vi "力特性判定.vi"(0 "曲线引用":refnum<vi>, 1 "力特性判定条件":T1, 3 "错误输入":errorcluster) -> (7 "曲线引用输出":refnum<vi>, 8 "OK？":bool, 10 "错误输出":errorcluster)   [LabVIEW 2020]
uses:
  Global_Variable/A131258.vi
  Global_Variable/Global.vi
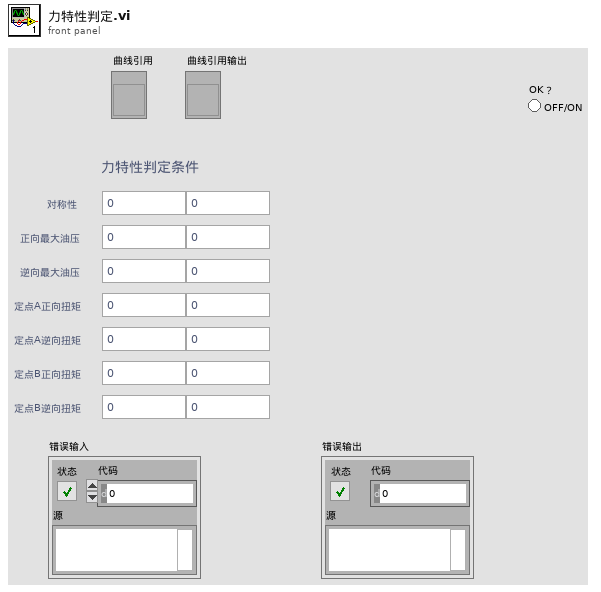
[diagram p1: front panel]
types:
  T1 = cluster{"           对称性":cluster{"下限":dbl, "上限":dbl}, "  正向最大油压":cluster{"下限":dbl, "上限":dbl}, "  逆向最大油压":cluster{"下限":dbl, "上限":dbl}, "定点A正向扭矩":cluster{"下限":dbl, "上限":dbl}, "定点A逆向扭矩":cluster{"下限":dbl, "上限":dbl}, "定点B正向扭矩":cluster{"下限":dbl, "上限":dbl}, "定点B逆向扭矩":cluster{"下限":dbl, "上限":dbl}}
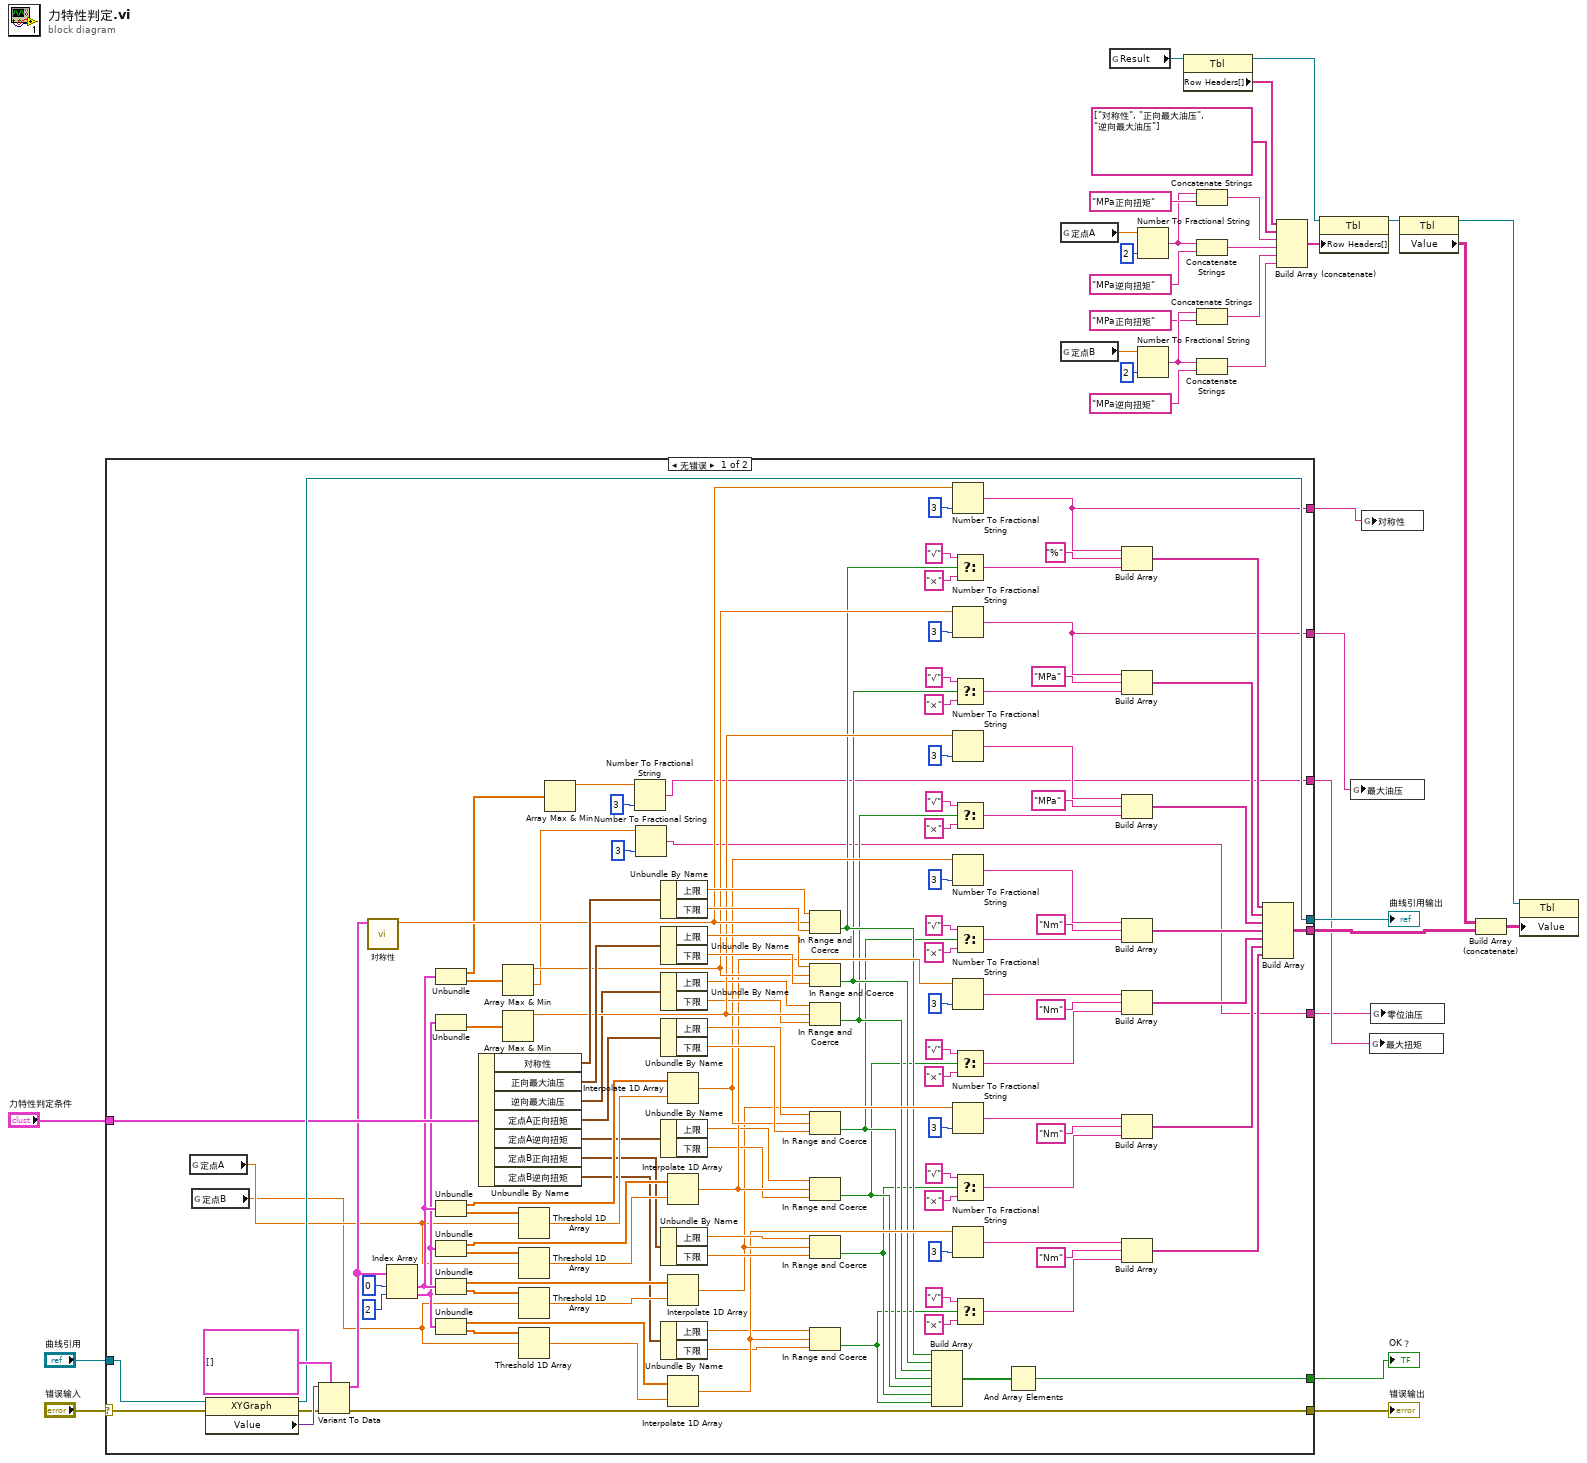
[diagram p0: block diagram]
diagram:
  n1 = case shown="无错误" "错误输入" {
    selector: "错误输入" -> [w155 w159]
    tunnel: [w152 w159] -> w33
    tunnel: "曲线引用" -> [w151 w158]
    tunnel: [w154 w158] -> w31
    tunnel: [w49 _] -> w30
    tunnel: "力特性判定条件" -> [w150 _]
    tunnel: [w48 _] -> w25
    tunnel: [w43 _] -> w4
    tunnel: [w42 _] -> w3
    tunnel: [w38 _] -> w2
    tunnel: [w35 _] -> w1
    frame No Error {
      n2 = global read "A131258.vi" "定点A"() -> (w45:dbl)
      n3 = global read "A131258.vi" "定点B"() -> (w44:dbl)
      n4 = property class="XYGraph"(reference=w151, error in=w155) -> (reference out=w154:refnum<vi>, error out=w153:errorcluster, "Value"=w157:variant)
      n5 = Variant To Data(error in=w153, type=cluster{dbl[], dbl[]}[] [], Variant=w157) -> (data=w140:cluster{dbl[], dbl[]}[], error out=w152:errorcluster)
      n6 = call "对称性.vi"("XY图"=w140) -> ("对称性"=w146:dbl)  [unwired: 10 in]
      n7 = Index Array(array=w140, index #1=0 ("索引"), index #2=2 ("索引")) -> (element #1=w79:cluster{dbl[], dbl[]}, element #2=w66:cluster{dbl[], dbl[]})
      n8 = Unbundle(w79) -> (w41:dbl[], w47:dbl[])
      n9 = Unbundle(w66) -> (w46:dbl[])  [unwired: 1 out]
      n10 = Unbundle(w79) -> (w111:dbl[], w112:dbl[])
      n11 = Unbundle(w66) -> (w105:dbl[], w104:dbl[])
      n12 = Unbundle(w79) -> (w85:dbl[], w86:dbl[])
      n13 = Unbundle(w66) -> (w76:dbl[], w75:dbl[])
      n14 = Unbundle By Name(w150) -> ("对称性"=w149:cluster{"下限":dbl, "上限":dbl}, "正向最大油压"=w132:cluster{"下限":dbl, "上限":dbl}, "逆向最大油压"=w121:cluster{"下限":dbl, "上限":dbl}, "定点A正向扭矩"=w108:cluster{"下限":dbl, "上限":dbl}, "定点A逆向扭矩"=w95:cluster{"下限":dbl, "上限":dbl}, "定点B正向扭矩"=w80:cluster{"下限":dbl, "上限":dbl}, "定点B逆向扭矩"=w65:cluster{"下限":dbl, "上限":dbl})
      n15 = Array Max & Min(array=w47) -> (max value=w131:dbl, min value=w36:dbl)  [unwired: 2 out]
      n16 = Array Max & Min(array=w46) -> (max value=w130:dbl)  [unwired: 3 out]
      n17 = Threshold 1D Array(2:w45, 3:w112) -> (0:w110:dbl)  [unwired: 1 in]
      n18 = Threshold 1D Array(2:w45, 3:w104) -> (0:w106:dbl)  [unwired: 1 in]
      n19 = Threshold 1D Array(2:w44, 3:w86) -> (0:w84:dbl)  [unwired: 1 in]
      n20 = Threshold 1D Array(2:w44, 3:w75) -> (0:w77:dbl)  [unwired: 1 in]
      n21 = Array Max & Min(array=w41) -> (max value=w39:dbl)  [unwired: 3 out]
      n22 = Number To Fractional String(number=w39, precision (6)=i16 3 ("精度(6)")) -> (F-format string=w38:string)  [unwired: 2 in]
      n23 = Number To Fractional String(number=w36, precision (6)=i16 3 ("精度(6)")) -> (F-format string=w35:string)  [unwired: 2 in]
      n24 = Unbundle By Name(w149) -> ("上限"=w148:dbl, "下限"=w147:dbl)
      n25 = Unbundle By Name(w132) -> ("上限"=w133:dbl, "下限"=w134:dbl)
      n26 = Unbundle By Name(w121) -> ("上限"=w129:dbl, "下限"=w128:dbl)
      n27 = Unbundle By Name(w108) -> ("上限"=w113:dbl, "下限"=w114:dbl)
      n28 = Unbundle By Name(w95) -> ("上限"=w103:dbl, "下限"=w102:dbl)
      n29 = Unbundle By Name(w80) -> ("上限"=w87:dbl, "下限"=w88:dbl)
      n30 = Unbundle By Name(w65) -> ("上限"=w74:dbl, "下限"=w73:dbl)
      n31 = Interpolate 1D Array(1:w110, 2:w111) -> (0:w109:dbl)
      n32 = Interpolate 1D Array(1:w106, 2:w105) -> (0:w107:dbl)
      n33 = Interpolate 1D Array(1:w84, 2:w85) -> (0:w83:dbl)
      n34 = Interpolate 1D Array(1:w77, 2:w76) -> (0:w78:dbl)
      n35 = In Range and Coerce(upper limit=w148, x=w146, lower limit=w147) -> (In Range?=w63:bool)  [unwired: 1 out]
      n36 = In Range and Coerce(upper limit=w133, x=w131, lower limit=w134) -> (In Range?=w61:bool)  [unwired: 1 out]
      n37 = In Range and Coerce(upper limit=w129, x=w130, lower limit=w128) -> (In Range?=w59:bool)  [unwired: 1 out]
      n38 = In Range and Coerce(upper limit=w113, x=w109, lower limit=w114) -> (In Range?=w57:bool)  [unwired: 1 out]
      n39 = In Range and Coerce(upper limit=w103, x=w107, lower limit=w102) -> (In Range?=w55:bool)  [unwired: 1 out]
      n40 = In Range and Coerce(upper limit=w87, x=w83, lower limit=w88) -> (In Range?=w53:bool)  [unwired: 1 out]
      n41 = In Range and Coerce(upper limit=w74, x=w78, lower limit=w73) -> (In Range?=w51:bool)  [unwired: 1 out]
      n42 = Build Array(w63, w61, w59, w57, w55, w53, w51) -> (w50:bool[])
      n43 = Number To Fractional String(number=w146, precision (6)=i16 3 ("精度(6)")) -> (F-format string=w43:string)  [unwired: 2 in]
      n44 = Number To Fractional String(number=w131, precision (6)=i16 3 ("精度(6)")) -> (F-format string=w42:string)  [unwired: 2 in]
      n45 = Number To Fractional String(number=w130, precision (6)=i16 3 ("精度(6)")) -> (F-format string=w126:string)  [unwired: 2 in]
      n46 = Number To Fractional String(number=w109, precision (6)=i16 3 ("精度(6)")) -> (F-format string=w116:string)  [unwired: 2 in]
      n47 = Number To Fractional String(number=w107, precision (6)=i16 3 ("精度(6)")) -> (F-format string=w100:string)  [unwired: 2 in]
      n48 = Number To Fractional String(number=w83, precision (6)=i16 3 ("精度(6)")) -> (F-format string=w90:string)  [unwired: 2 in]
      n49 = Number To Fractional String(number=w78, precision (6)=i16 3 ("精度(6)")) -> (F-format string=w71:string)  [unwired: 2 in]
      n50 = Select(t="√" ("元素"), s=w63, f="×" ("元素")) -> (s? t:f=w141:string)
      n51 = Select(t="√" ("元素"), s=w61, f="×" ("元素")) -> (s? t:f=w139:string)
      n52 = Select(t="√" ("元素"), s=w59, f="×" ("元素")) -> (s? t:f=w122:string)
      n53 = Select(t="√" ("元素"), s=w57, f="×" ("元素")) -> (s? t:f=w120:string)
      n54 = Select(t="√" ("元素"), s=w55, f="×" ("元素")) -> (s? t:f=w96:string)
      n55 = Select(t="√" ("元素"), s=w53, f="×" ("元素")) -> (s? t:f=w94:string)
      n56 = Select(t="√" ("元素"), s=w51, f="×" ("元素")) -> (s? t:f=w67:string)
      n57 = And Array Elements(Boolean array=w50) -> (logical AND=w49:bool)
      n58 = Build Array(w43, "%" ("元素"), w141) -> (w64:string[])
      n59 = Build Array(w42, "MPa" ("元素"), w139) -> (w62:string[])
      n60 = Build Array(w126, "MPa" ("元素"), w122) -> (w60:string[])
      n61 = Build Array(w116, "Nm" ("元素"), w120) -> (w58:string[])
      n62 = Build Array(w100, "Nm" ("元素"), w96) -> (w56:string[])
      n63 = Build Array(w90, "Nm" ("元素"), w94) -> (w54:string[])
      n64 = Build Array(w71, "Nm" ("元素"), w67) -> (w52:string[])
      n65 = Build Array(w64, w62, w60, w58, w56, w54, w52) -> (w48:string[][])
    }
    frame Error {
    }
  }
  "错误输出" <- w33
  "曲线引用输出" <- w31
  "OK？" <- w30
  n66 = global read "A131258.vi" "定点A"() -> (w18:dbl)
  n67 = global read "A131258.vi" "定点B"() -> (w17:dbl)
  n68 = global read "Global.vi" "Result"() -> (w24:refnum<vi>)
  n69 = Number To Fractional String(number=w18, precision (6)=i16 2 ("精度(6)")) -> (F-format string=w15:string)  [unwired: 2 in]
  n70 = Number To Fractional String(number=w17, precision (6)=i16 2 ("精度(6)")) -> (F-format string=w12:string)  [unwired: 2 in]
  n71 = property class="Tbl"(reference=w24) -> (reference out=w23:refnum<vi>, "Row Headers[]"=w21:string[])  [unwired: 1 in, 1 out]
  n72 = Concatenate Strings(w15, "MPa正向扭矩") -> (w10:string)
  n73 = Concatenate Strings(w15, "MPa逆向扭矩") -> (w9:string)
  n74 = Concatenate Strings(w12, "MPa正向扭矩") -> (w8:string)
  n75 = Concatenate Strings(w12, "MPa逆向扭矩") -> (w7:string)
  n76 = Build Array (concatenate)(w21, string[] ["对称性", "正向最大油压", "逆向最大油压"] ("列首字符串[]"), w10, w9, w8, w7) -> (w19:string[])
  n77 = property class="Tbl"(reference=w23, "Row Headers[]"=w19) -> (reference out=w22:refnum<vi>)  [unwired: 1 in, 1 out]
  n78 = global write "检测结果.vi" "最大油压"(w3) -> ()
  n79 = global write "检测结果.vi" "对称性"(w4) -> ()
  n80 = global write "检测结果.vi" "最大扭矩"(w2) -> ()
  n81 = global write "检测结果.vi" "零位油压"(w1) -> ()
  n82 = property class="Tbl"(reference=w22) -> (reference out=w28:refnum<vi>, "Value"=w27:string[][])  [unwired: 1 in, 1 out]
  n83 = Build Array (concatenate)(w27, w25) -> (w26:string[][])
  n84 = property class="Tbl"(reference=w28, "Value"=w26) -> ()  [unwired: 1 in, 2 out]
